vi "PerformMeasurements.vi"() -> ()   [LabVIEW 2017]
panel:
  in  "Stop Measurement":bool
  in  "Measurement Interval [s]":i32
  out "?":dbl
  out "?":dbl
  out "Humidity":dbl(graph)
  out "Temperature":dbl(graph)
  out "Error Monitor":errorcluster
  out "Humidity [%]":dbl(slide) scale=20.0..90.0
  out "Temperature [C]":dbl(slide) scale=15.0..30.0
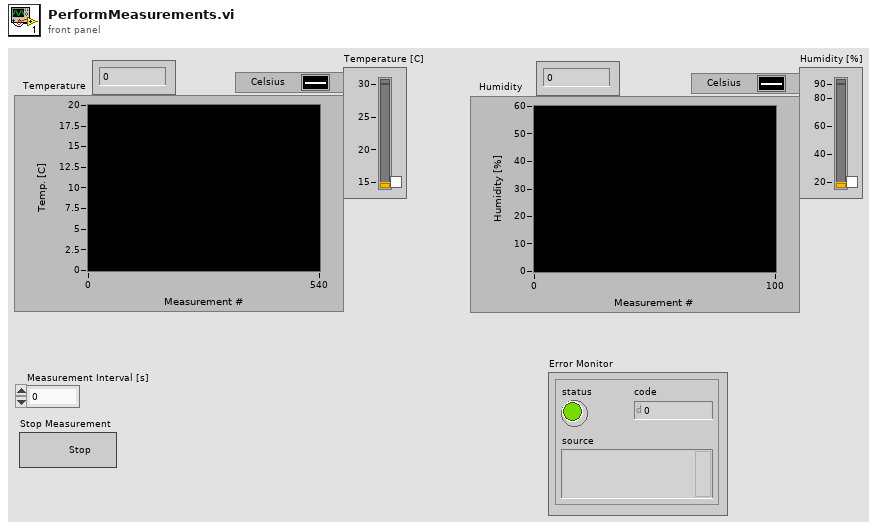
[diagram p1: front panel]
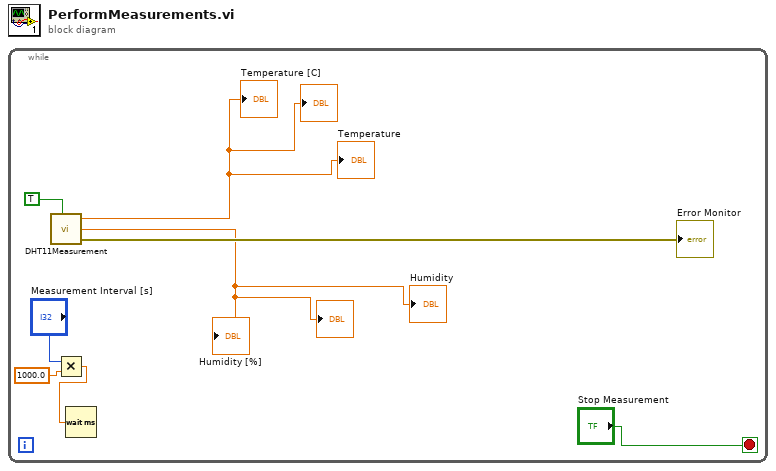
[diagram p0: block diagram]
diagram:
  n1 = while {
    stop <- "Stop Measurement" stop-if-true
    n2 = call "DHT11Measurement.vi"("Perform Measurement"=TRUE) -> ("Temperature (C)"=→"Temperature [C]" →"Temperature" →"?":dbl, "Humidity (%)"=→"Humidity [%]" →"Humidity" →"?":dbl, "error out"=→"Error Monitor":errorcluster)  [unwired: 5 in]
    n3 = Multiply(x="Measurement Interval [s]", y=1000.0) -> (x*y=w2:dbl)
    n4 = Wait (ms)(milliseconds to wait=w2) -> ()  [unwired: 1 out]
  }
